vi "TAT_Varient Creater.vi"(8 "error in (no error)":errorcluster) -> (0 "error out":errorcluster)   [LabVIEW 2017]
uses:
  <vilib>/Utility/config.llb/Read Key (I32).vi
  <vilib>/Utility/config.llb/Write Key (U32).vi
  <vilib>/Utility/config.llb/NI_LVConfig.lvlib
panel:
  in  "Delete Square":bool
  in  "EDIT & SAVE":bool
  in  "Varient Details":string[][](table)
  in  "BATCH SIZE":u16=1 min=1 max=100 step=1
  in  "VARIENT NUMBER":u16=1 min=1 max=100 step=1
  in  "HOME":bool
  in  "UPDATE TABLE":bool
  in  "VARIENT NAME":string(combo)
  # "Varient Creater"
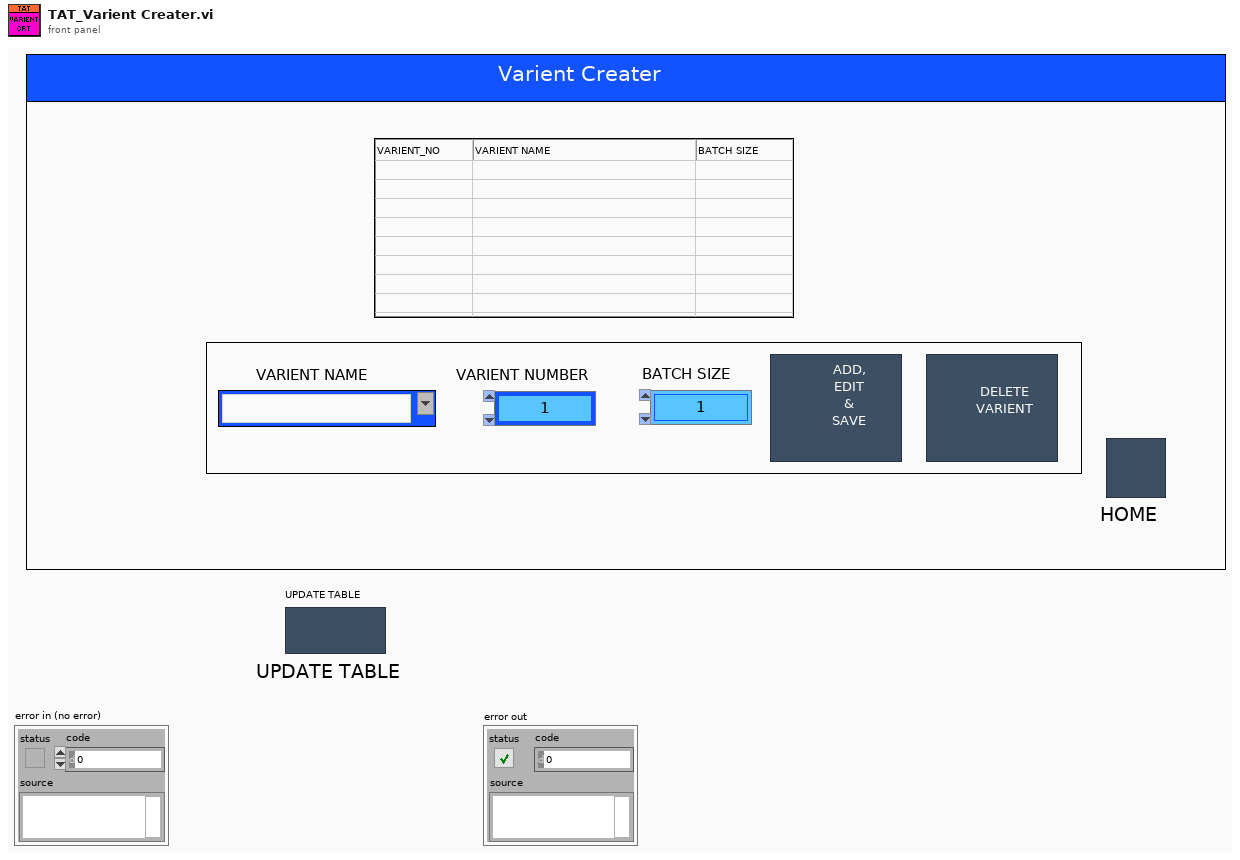
[diagram p1: front panel]
types:
  T1 = enum32{"invalid app kind", "Development System", "Run Time System", "Student Edition", "Embedded LabVIEW", "Evaluation", "Custom"}
  T2 = typedef "NI_LVConfig.lvlib/Config Data RefNum.ctl" = refnum<k1>
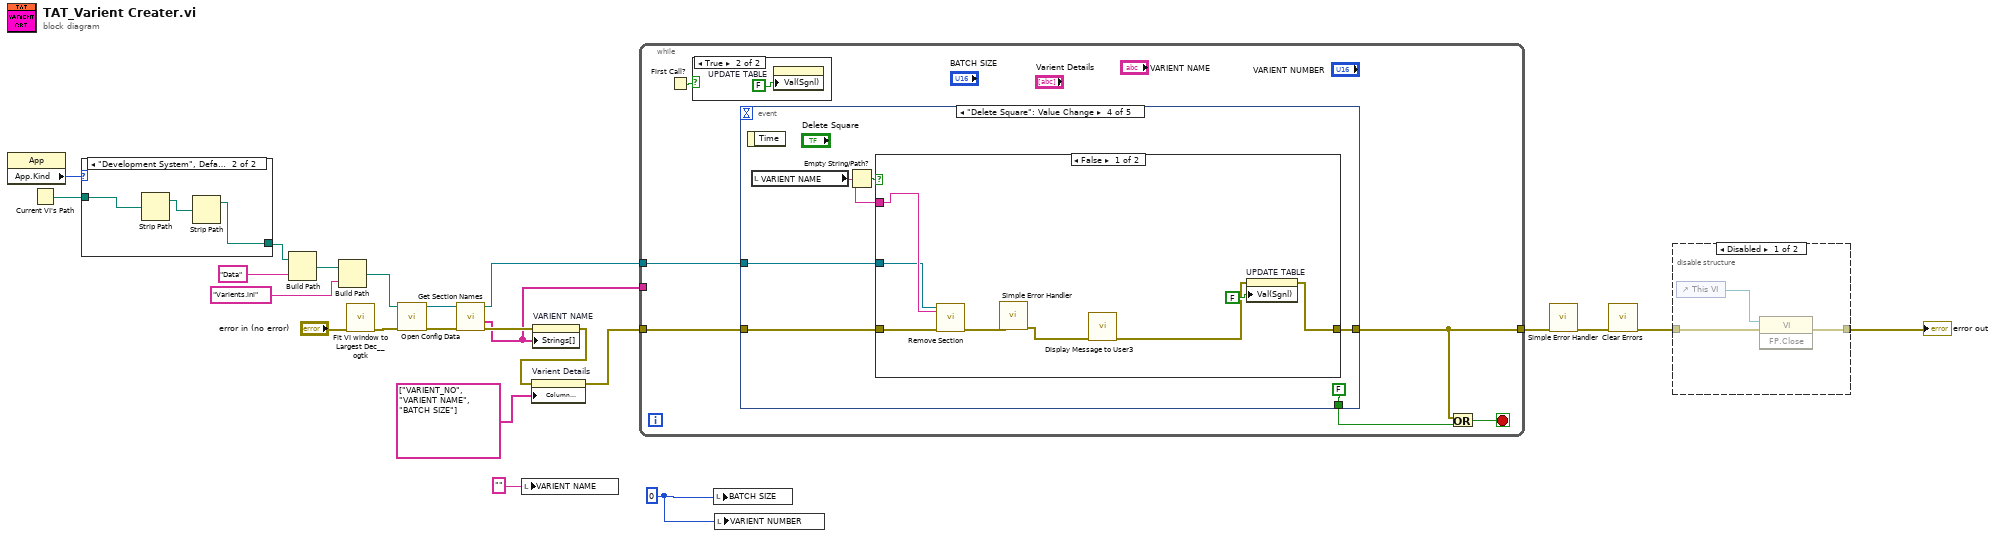
[diagram p0: block diagram]
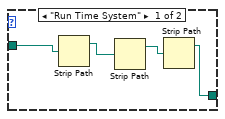
[diagram p3: hidden frame]
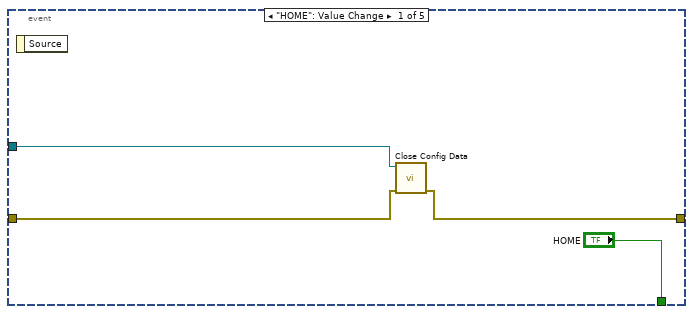
[diagram p5: hidden frame]
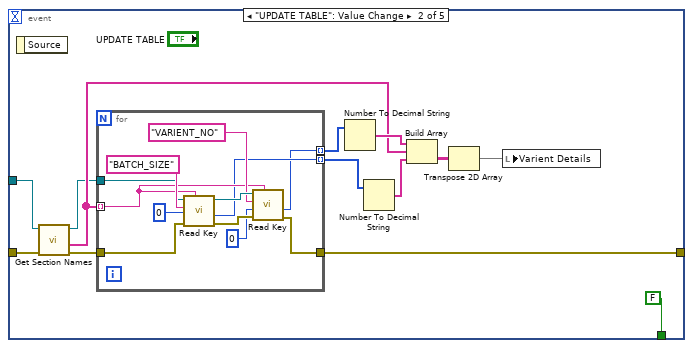
[diagram p6: hidden frame]
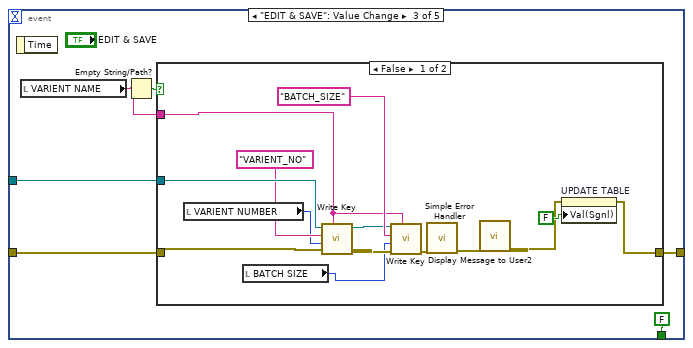
[diagram p7: hidden frame]
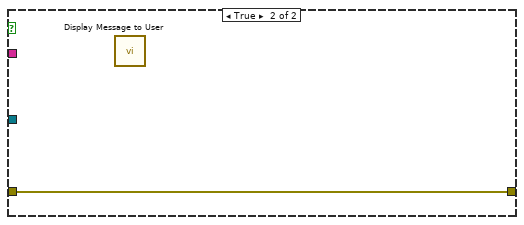
[diagram p8: hidden frame]
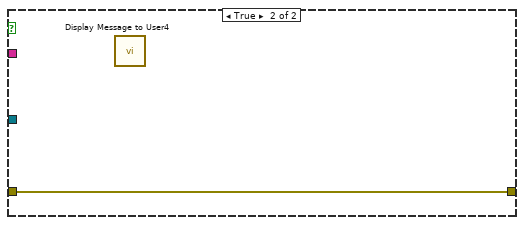
[diagram p9: hidden frame]
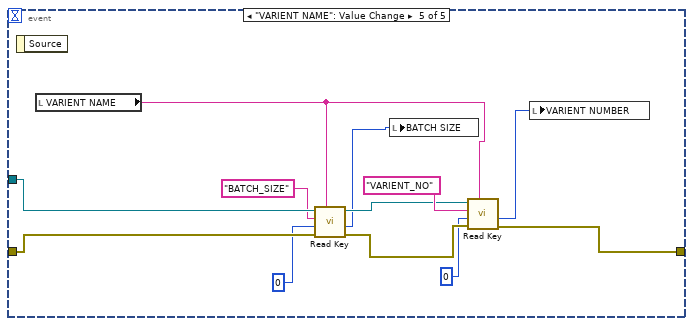
[diagram p10: hidden frame]
diagram:
  w1 = 0 ("default value")
  n1 = property class="App"() -> ("App.Kind"=w18:T1)  [unwired: 2 in, 2 out]
  n2 = Current VI's Path() -> (path=w19:path)
  n3 = case shown="\"Development System\", Default" w18 {
    tunnel: w19 -> [w25 w29]
    tunnel: [w24 w28] -> w16
    frame "Run Time System" {
      n4 = Strip Path(path=w25) -> (stripped path=w27:path)  [unwired: 1 out]
      n5 = Strip Path(path=w27) -> (stripped path=w26:path)  [unwired: 1 out]
      n6 = Strip Path(path=w26) -> (stripped path=w24:path)  [unwired: 1 out]
    }
    frame "Development System", Default {
      n7 = Strip Path(path=w29) -> (stripped path=w30:path)  [unwired: 1 out]
      n8 = Strip Path(path=w30) -> (stripped path=w28:path)  [unwired: 1 out]
    }
  }
  n9 = Build Path(base path=w16, name or relative path="Data") -> (appended path=w17:path)
  n10 = Build Path(base path=w17, name or relative path="Varients.ini") -> (appended path=w15:path)
  n11 = call <userlib>:"Fit VI window to Largest Dec__ogtk.vi"("error in (no error)"="error in (no error)") -> ("error out"=w9:errorcluster)  [unwired: 5 in, 1 out]
  n12 = call <vilib>:"Open Config Data.vi"("error in (no error)"=w9, "configuration file path"=w15) -> ("error out"=w11:errorcluster, "refnum"=w12:T2)  [unwired: 7 in, 1 out]
  n13 = call <vilib>:"Get Section Names.vi"("error in (no error)"=w11, "refnum"=w12) -> ("error out"=w10:errorcluster, "section names"=w3:string[], "refnum out"=w7:T2)  [unwired: 7 in]
  n14 = local write "VARIENT NAME"("" ("name or relative path")) -> ()
  n15 = property on="VARIENT NAME" class="CmbBox"(error in=w10, "Strings[]"=w3) -> (error out=w6:errorcluster)  [unwired: 1 in, 1 out]
  n16 = property on="Varient Details" class="Tbl (strict)"(error in=w6, "Column Headers[]"=string[] ["VARIENT_NO", "VARIENT NAME", "BATCH SIZE"] ("Column Header Strings[]")) -> (error out=w5:errorcluster)  [unwired: 1 in, 1 out]
  n17 = while {
    tunnel: w5 -> [w35]
    tunnel: [w33] -> w20
    tunnel: w7 -> [w32]
    tunnel: w3 -> [_]
    stop <- w34 stop-if-true
    n18 = First Call?() -> (First Call?: T/F=w31:bool)
    n19 = case shown="True" w31 {
      frame False {
      }
      frame True {
        n20 = property on="UPDATE TABLE" class="Bool (strict)"("Val(Sgnl)"=FALSE) -> ()  [unwired: 2 in, 2 out]
      }
    }
    n21 = event shown="[3] \"Delete Square\": Value Change" {
      selector: _ -> [_ _ _ _ _]
      dyn-events: _ -> [_ _ _ _ _]
      timeout: _ -> [_ _ _ _ _]
      tunnel: ["HOME" FALSE ("stop") FALSE ("stop") FALSE ("stop") _] -> w36
      tunnel: w35 -> [w40 w46 w68 w89 w114]
      tunnel: [w39 w53 w71 w92 w109] -> w33
      tunnel: w32 -> [w38 w43 w69 w90 w113]
      event "HOME": Value Change {
        n22 = event-data() -> ()  [unwired: 1 in, 1 out]
        n23 = call <vilib>:"Close Config Data.vi"("error in (no error)"=w40, "refnum"=w38) -> ("error out"=w39:errorcluster)  [unwired: 8 in, 1 out]
      }
      event "UPDATE TABLE": Value Change {
        n24 = event-data() -> ()  [unwired: 1 in, 1 out]
        n25 = call <vilib>:"Get Section Names.vi"("error in (no error)"=w46, "refnum"=w43) -> ("error out"=w45:errorcluster, "section names"=w44:string[], "refnum out"=w42:T2)  [unwired: 7 in]
        n26 = for {
          tunnel: [w60] -> w53
          tunnel: w45 -> [w59]
          tunnel: w44 -> [w58] mode=indexing
          tunnel: w42 -> [w57]
          tunnel: [w56] -> w51 mode=indexing
          tunnel: [w55] -> w52 mode=indexing
          n27 = call-poly <vilib>:"Read Key.vi"("section"=w58, "error in (no error)"=w59, "default value"=0, "key"="BATCH_SIZE", "refnum"=w57) -> ("error out"=w66:errorcluster, "value"=w56:i32, "refnum out"=w65:T2)  [unwired: 3 in, 1 out]
          n28 = call-poly <vilib>:"Read Key.vi"("section"=w58, "error in (no error)"=w66, "default value"=0, "key"="VARIENT_NO", "refnum"=w65) -> ("error out"=w60:errorcluster, "value"=w55:i32)  [unwired: 3 in, 2 out]
        }
        n29 = Number To Decimal String(number=w52) -> (decimal integer string=w47:string[])  [unwired: 1 in]
        n30 = Number To Decimal String(number=w51) -> (decimal integer string=w50:string[])  [unwired: 1 in]
        n31 = Build Array(w47, w44, w50) -> (w49:string[][])
        n32 = Transpose 2D Array(2D array=w49) -> (transposed array=w48:string[][])
        n33 = local write "Varient Details"(w48) -> ()
      }
      event "EDIT & SAVE": Value Change {
        n34 = event-data() -> ()  [unwired: 1 in, 1 out]
        n35 = local read "VARIENT NAME"() -> (w67:string)
        n36 = Empty String/Path?(string/path=w67) -> (empty?=w70:bool)
        n37 = case shown="False" w70 {
          tunnel: w68 -> [w85 w87]
          tunnel: [w78 w87] -> w71
          tunnel: w69 -> [w83 _]
          tunnel: w67 -> [w80 _]
          frame False {
            n38 = local read "VARIENT NUMBER"() -> (w76:u16)
            n39 = local read "BATCH SIZE"() -> (w77:u16)
            n40 = call-poly <vilib>:"Write Key.vi"("section"=w80, "error in (no error)"=w85, "value"=w76, "key"="VARIENT_NO", "refnum"=w83) -> ("error out"=w84:errorcluster, "refnum out"=w82:T2)  [unwired: 4 in, 1 out]
            n41 = call-poly <vilib>:"Write Key.vi"("section"=w80, "error in (no error)"=w84, "value"=w77, "key"="BATCH_SIZE", "refnum"=w82) -> ("error out"=w75:errorcluster)  [unwired: 4 in, 2 out]
            n42 = call <vilib>:"Simple Error Handler.vi"("error in (no error)"=w75) -> ("error out"=w74:errorcluster)  [unwired: 4 in, 4 out]
            n43 = call "Display Message to User2"("error in (no error)"=w74) -> ("error out"=w73:errorcluster)  [unwired: 9 in, 1 out]
            n44 = property on="UPDATE TABLE" class="Bool (strict)"(error in=w73, "Val(Sgnl)"=FALSE) -> (error out=w78:errorcluster)  [unwired: 1 in, 1 out]
          }
          frame True {
            n45 = call "Display Message to User"() -> ()  [unwired: 10 in, 2 out]
          }
        }
      }
      event "Delete Square": Value Change {
        n46 = event-data() -> ()  [unwired: 1 in, 1 out]
        n47 = local read "VARIENT NAME"() -> (w88:string)
        n48 = Empty String/Path?(string/path=w88) -> (empty?=w91:bool)
        n49 = case shown="False" w91 {
          tunnel: w89 -> [w95 w102]
          tunnel: [w100 w102] -> w92
          tunnel: w90 -> [w96 _]
          tunnel: w88 -> [w97 _]
          frame False {
            n50 = call <vilib>:"Remove Section.vi"("section"=w97, "error in (no error)"=w95, "refnum"=w96) -> ("error out"=w94:errorcluster)  [unwired: 6 in, 2 out]
            n51 = call <vilib>:"Simple Error Handler.vi"("error in (no error)"=w94) -> ("error out"=w99:errorcluster)  [unwired: 4 in, 4 out]
            n52 = call "Display Message to User3"("error in (no error)"=w99) -> ("error out"=w98:errorcluster)  [unwired: 9 in, 1 out]
            n53 = property on="UPDATE TABLE" class="Bool (strict)"(error in=w98, "Val(Sgnl)"=FALSE) -> (error out=w100:errorcluster)  [unwired: 1 in, 1 out]
          }
          frame True {
            n54 = call "Display Message to User4"() -> ()  [unwired: 10 in, 2 out]
          }
        }
      }
      event "VARIENT NAME": Value Change {
        n55 = event-data() -> ()  [unwired: 1 in, 1 out]
        n56 = local read "VARIENT NAME"() -> (w103:string)
        n57 = call-poly <vilib>:"Read Key.vi"("section"=w103, "error in (no error)"=w114, "default value"=0, "key"="BATCH_SIZE", "refnum"=w113) -> ("error out"=w110:errorcluster, "value"=w104:i32, "refnum out"=w108:T2)  [unwired: 3 in, 1 out]
        n58 = local write "BATCH SIZE"(w104) -> ()
        n59 = call-poly <vilib>:"Read Key.vi"("section"=w103, "error in (no error)"=w110, "default value"=0, "key"="VARIENT_NO", "refnum"=w108) -> ("error out"=w109:errorcluster, "value"=w107:i32)  [unwired: 3 in, 2 out]
        n60 = local write "VARIENT NUMBER"(w107) -> ()
      }
    }
    n61 = Or(x=w33, y=w36) -> (x .or. y?=w34:bool)
  }
  n62 = local write "BATCH SIZE"(w1) -> ()
  n63 = local write "VARIENT NUMBER"(w1) -> ()
  n64 = call <vilib>:"Simple Error Handler.vi"("error in (no error)"=w20) -> ("error out"=w23:errorcluster)  [unwired: 4 in, 4 out]
  n65 = call <vilib>:"Clear Errors.vi"("error in (no error)"=w23) -> ("error out"=w22:errorcluster)  [unwired: 5 in, 1 out]
  n66 = disable-structure shown="Disabled" {
    disable-tunnel: w22 -> [w117 w118]
    disable-tunnel: [w116 w118] -> w21
    frame Disabled {
      n67 = control-ref of="This VI"() -> (w115:refnum<vi>)
      n68 = invoke class="VI" method="FP.Close"(reference=w115, error in=w117) -> (error out=w116:errorcluster)  [unwired: 1 in, 2 out]
    }
    frame Enabled {
    }
  }
  "error out" <- w21
